vi "Target Centralization.vi"(2 "Current angle X":dbl, 3 "Traget position X":dbl, 4 "Current angle Y":dbl, 5 "Traget position Y":dbl) -> (0 "The Angle Set Point X":dbl, 1 "The Angle Set Point Y":dbl)   [LabVIEW 2012]
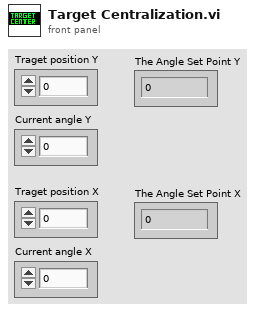
[diagram p1: front panel]
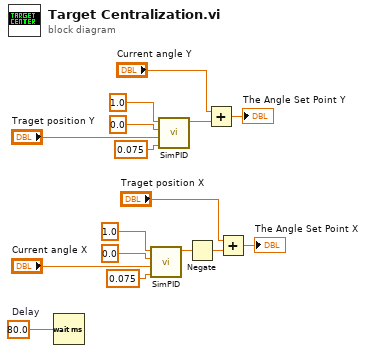
[diagram p0: block diagram]
diagram:
  w14 = 80.0  # Delay
  n1 = Wait (ms)(milliseconds to wait=w14) -> ()  [unwired: 1 out]
  n2 = call "SimPID.vi"("Range"=0.075, "Position"="Current angle X", "Set Point"=0.0, "Gain"=1.0 ("Set Point")) -> ("result"=w5:dbl)  [unwired: 5 in, 1 out]
  n3 = call "SimPID.vi"("Range"=0.075, "Position"="Traget position Y", "Set Point"=0.0, "Gain"=1.0 ("Set Point")) -> ("result"=w16:dbl)  [unwired: 5 in, 1 out]
  n4 = Negate(x=w5) -> (-x=w1:dbl)
  n5 = Add(x="Current angle Y", y=w16) -> (x+y=→"The Angle Set Point Y":dbl)
  n6 = Add(x="Traget position X", y=w1) -> (x+y=→"The Angle Set Point X":dbl)
